vi "np_astype_str.vi"(11 "NG_rules":dbl[](array[numeric])) -> (3 "Array":string[](array[string]))   [LabVIEW 2017]
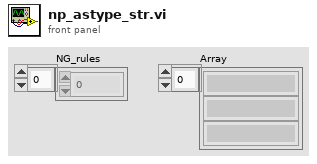
[diagram p1: front panel]
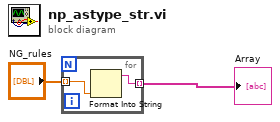
[diagram p0: block diagram]
diagram:
  n1 = for {
    tunnel: "NG_rules" -> [w3] mode=indexing
    tunnel: [w4] -> w2 mode=indexing
    n2 = Format Into String(w3) -> (resulting string=w4:string)  [unwired: 3 in, 1 out]
  }
  "Array" <- w2
